vi "Setup.vi"(8 "Error In":errorcluster, 9 "Password":string, 10 "Username":string, 11 "Address":string) -> (0 "Error Out":errorcluster, 3 "Agent":refnum<class "Agent.lvclass">)   [LabVIEW 2018, in "Tests.lvlib" / "Agent.lvlib"]
uses:
  Agent.lvlib
  src/Toolkit/Agent/Agent.lvclass
  src/Toolkit/Session/Support/Create from SSH.vi
  src/Toolkit/Session/Support/Password Authentication.vi
  src/Toolkit/Agent/Support/Create from Session.vi
  src/Toolkit/SSH/SSH.lvclass
  src/Toolkit/Session/Session.lvclass
  Tests.lvlib
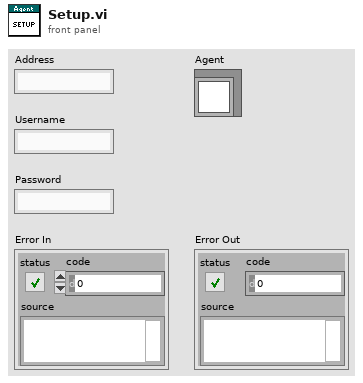
[diagram p1: front panel]
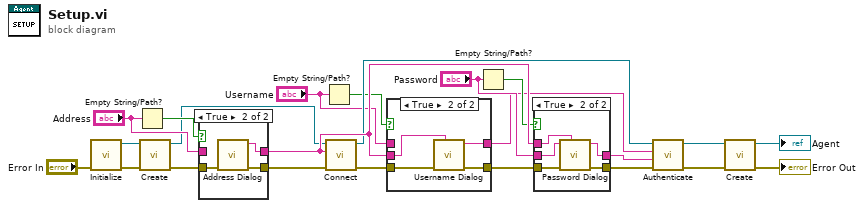
[diagram p0: block diagram]
diagram:
  n1 = call "Initialize.vi"("Error In"="Error In") -> ("Error Out"=w5:errorcluster, "SSH"=w6:refnum<class "SSH.lvclass">)  [unwired: 9 in]
  n2 = Empty String/Path?(string/path="Address") -> (empty?=w9:bool)
  n3 = call-poly "Create.vi"("Error In"=w5, "SSH"=w6) -> ("Error Out"=w11:errorcluster, "Sesssion"=w8:refnum<class "Session.lvclass">)  [unwired: 8 in]
  n4 = case shown="True" w9 {
    tunnel: w11 -> [w24 w28]
    tunnel: [w24 w27] -> w12
    tunnel: [w25 w26] -> w23
    tunnel: "Address" -> [w25 _]
    frame False {
    }
    frame True {
      n5 = call "Address Dialog.vi"("Error In"=w28) -> ("Error Out"=w27:errorcluster, "Address Out"=w26:string)  [unwired: 9 in]
    }
  }
  n6 = Empty String/Path?(string/path="Username") -> (empty?=w18:bool)
  n7 = call "Connect.vi"("Error In"=w12, "Address"=w23, "Session In"=w8) -> ("Error Out"=w21:errorcluster, "Sesssion Out"=w22:refnum<class "Session.lvclass">)  [unwired: 7 in]
  n8 = case shown="True" w18 {
    tunnel: w21 -> [w30 w34]
    tunnel: [w29 w33] -> w16
    tunnel: [w30 w32] -> w13
    tunnel: "Username" -> [w29 _]
    tunnel: w23 -> [_ w31]
    frame False {
    }
    frame True {
      n9 = call "Username Dialog.vi"("Address"=w31, "Error In"=w34) -> ("Error Out"=w32:errorcluster, "Username Out"=w33:string)  [unwired: 8 in]
    }
  }
  n10 = Empty String/Path?(string/path="Password") -> (empty?=w20:bool)
  n11 = case shown="True" w20 {
    tunnel: "Password" -> [w36 w41]
    tunnel: w13 -> [w35 w40]
    tunnel: [w35 w39] -> w14
    tunnel: [w36 w38] -> w15
    tunnel: w23 -> [_ w37]
    frame False {
    }
    frame True {
      n12 = call "Password Dialog.vi"("Address"=w37, "Error In"=w40, "Password In"=w41) -> ("Error Out"=w39:errorcluster, "Password Out"=w38:string)  [unwired: 7 in]
    }
  }
  n13 = call-poly "Authenticate.vi"("Error In"=w14, "Password"=w15, "Username"=w16, "Session In"=w22) -> ("Error Out"=w3:errorcluster, "Sesssion Out"=w4:refnum<class "Session.lvclass">)  [unwired: 6 in]
  n14 = call-poly "Create.vi"("Error In"=w3, "Session"=w4) -> ("Error Out"=→"Error Out":errorcluster, "Agent"=→"Agent":refnum<class "Agent.lvclass">)  [unwired: 8 in]
